vi "Unidenx and undbundle template.vi"() -> ()   [LabVIEW 2018]
panel:
  in  "Array":cluster{"Numeric":dbl}[](array[cluster])
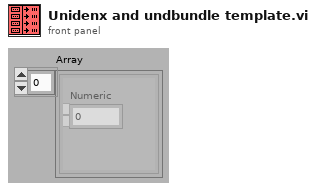
[diagram p1: front panel]
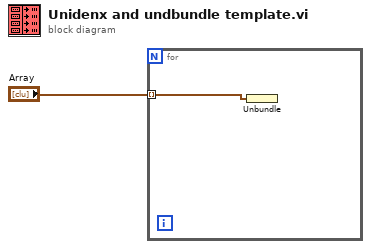
[diagram p0: block diagram]
diagram:
  n1 = for {
    tunnel: "Array" -> [w2] mode=indexing
    n2 = Unbundle(w2) -> ()  [unwired: 1 out]
  }
